vi "Two Backgate.vi"(0 "Sense":refnum<visa-resource-name>, 1 "Source":refnum<visa-resource-name>, 3 "Sense error in":errorcluster, 4 "Source error in":errorcluster, 6 "Input sweep":dbl[](array[numeric])) -> (8 "Read Time":dbl, 10 "BG Time Taken (s)":dbl, 11 "BackGate V":dbl[](array[numeric]), 12 "XY Graph":cluster{dbl[], "Ramp Pattern":dbl[]}(graph), 13 "Resistance":dbl[](array[numeric]), 14 "Sense Out":refnum<visa-resource-name>, 15 "Source Out":refnum<visa-resource-name>, 17 "Sense error out":errorcluster, 18 "Source error out":errorcluster)   [LabVIEW 2019, in "SMU.lvclass"]
uses:
  SMU.lvclass
  <instrlib>/Keithley 2450/Keithley 2450.lvlib
  <instrlib>/Keithley DMM6500 DAQ6500 Series/Keithley DMM6500 DAQ6500 Series.lvlib
panel:
  out "InitTime":dbl
  out "Total Time Taken (s) 2":dbl
  out "Sense Length":i32
  out "Current BG V":dbl
  out "Source buffer":string
  out "Current":dbl[](array[numeric])
  out "Voltage":dbl[](array[numeric])
  out "Sense buffer":string
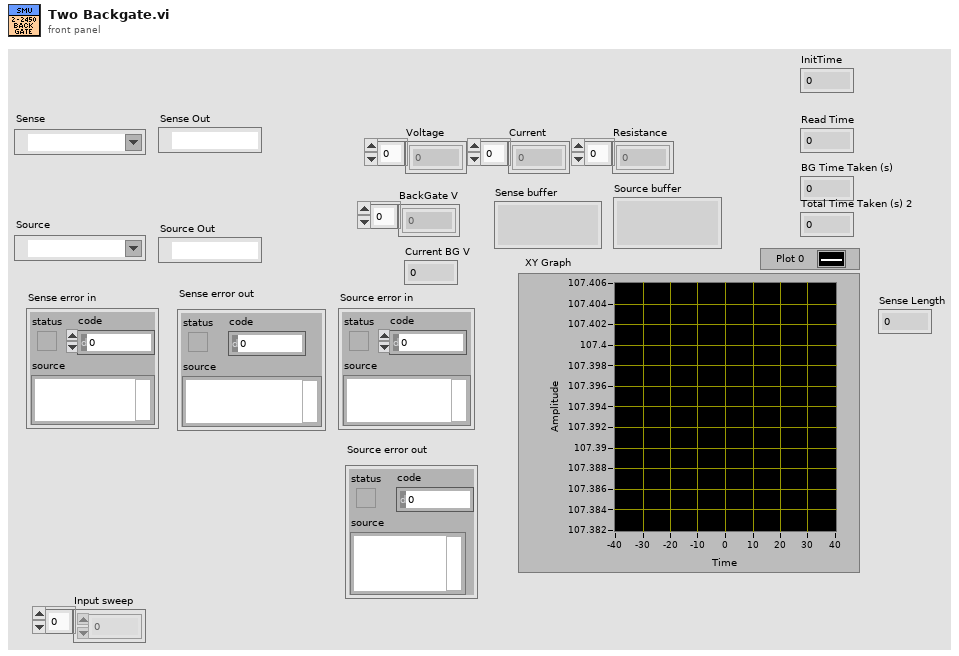
[diagram p1: front panel]
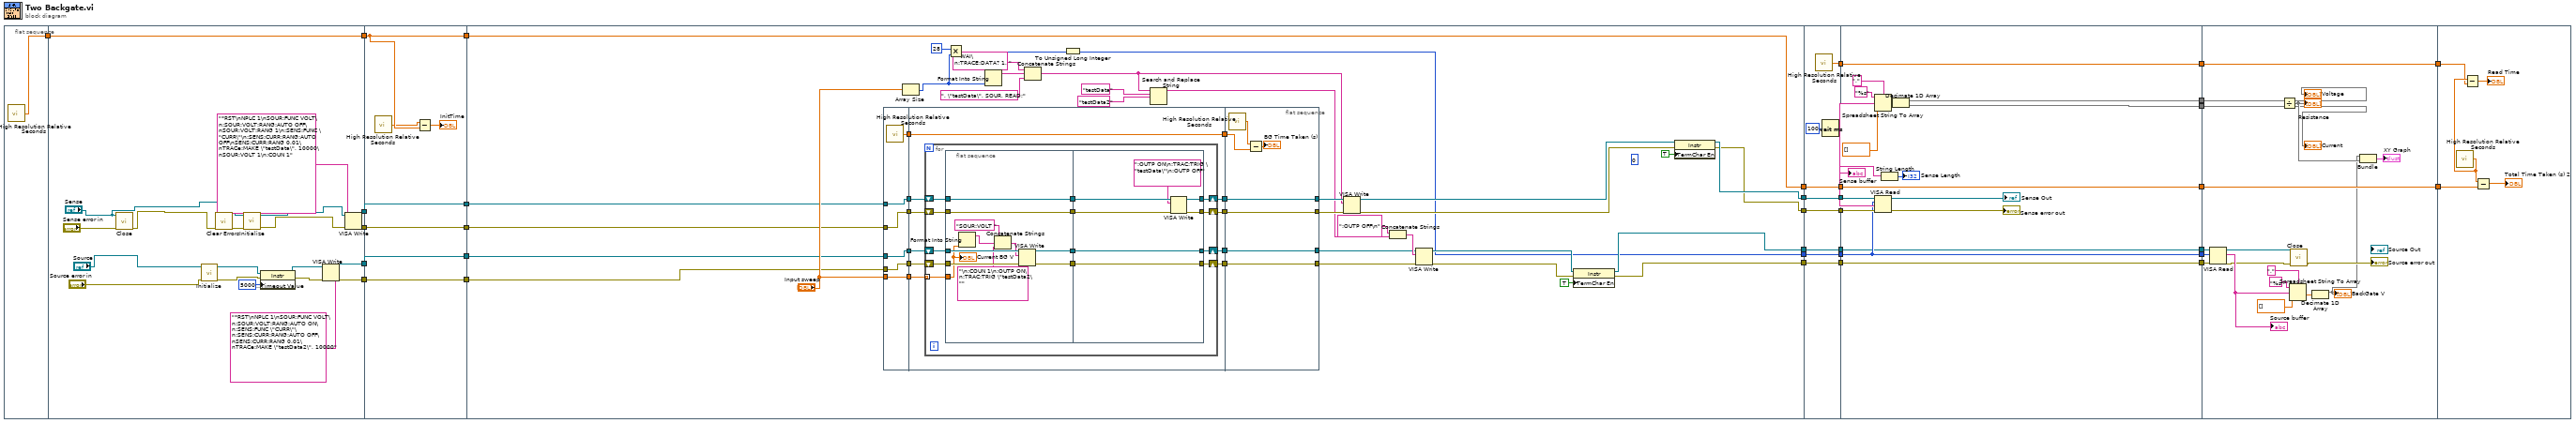
[diagram p0: block diagram]
diagram:
  n1 = flat-sequence {
    tunnel: [w34] -> w33
    tunnel: w33 -> [w54]
    tunnel: [w54] -> w20
    tunnel: [w41] -> w18
    tunnel: [w40] -> w16
    tunnel: [w39] -> w14
    tunnel: [w38] -> w12
    tunnel: w20 -> [w61]
    tunnel: [w61] -> w19
    tunnel: w18 -> [w60]
    tunnel: [w60] -> w17
    tunnel: w16 -> [w59]
    tunnel: [w59] -> w15
    tunnel: w14 -> [w58]
    tunnel: [w58] -> w13
    tunnel: w12 -> [w57]
    tunnel: [w57] -> w11
    tunnel: [w74] -> w32
    tunnel: w19 -> [w74]
    tunnel: w17 -> [w78]
    tunnel: w15 -> [w77]
    tunnel: w13 -> [w76]
    tunnel: w11 -> [w75]
    tunnel: [w63] -> w30
    tunnel: [w62] -> w28
    tunnel: [w64] -> w26
    tunnel: [w69] -> w23
    tunnel: [w68] -> w10
    tunnel: w32 -> [w167]
    tunnel: [w167] -> w31
    tunnel: w30 -> [w166]
    tunnel: [w166] -> w29
    tunnel: w28 -> [w165]
    tunnel: [w165] -> w27
    tunnel: w26 -> [w164]
    tunnel: [w164] -> w25
    tunnel: [w163] -> w24
    tunnel: w23 -> [w162]
    tunnel: [w162] -> w22
    tunnel: [w161] -> w21
    tunnel: w10 -> [w163]
    tunnel: w31 -> [w170]
    tunnel: [w170] -> w9
    tunnel: w29 -> [w175]
    tunnel: w27 -> [w174]
    tunnel: w25 -> [w173]
    tunnel: w24 -> [w179]
    tunnel: w22 -> [w178]
    tunnel: w21 -> [w176]
    tunnel: [w176] -> w7
    tunnel: [w175] -> w5
    tunnel: [w174] -> w4
    tunnel: [w173] -> w3
    tunnel: [w172] -> w2
    tunnel: [w171] -> w1
    tunnel: w9 -> [w202]
    tunnel: [w202] -> w8
    tunnel: w7 -> [w201]
    tunnel: [w201] -> w6
    tunnel: w5 -> [w194]
    tunnel: w4 -> [w193]
    tunnel: w3 -> [w192]
    tunnel: w2 -> [w188]
    tunnel: w1 -> [w187]
    tunnel: w8 -> [w206]
    tunnel: w6 -> [w204]
    frame #0 {
      n2 = call <vilib>:"High Resolution Relative Seconds.vi"() -> ("relative seconds"=w34:dbl)
    }
    frame #1 {
      n3 = call <instrlib>:"Close.vi"("error in (no error)"="Sense error in", "VISA resource name"="Sense") -> ("error out"=w47:errorcluster)  [unwired: 9 in]
      n4 = call <instrlib>:"Initialize.vi"("error in (no error)"="Source error in", "VISA resource name"="Source") -> ("error out"=w53:errorcluster, "VISA resource name out"=w50:refnum<visa-resource-name>)  [unwired: 8 in]
      n5 = call <vilib>:"Clear Errors.vi"("error in (no error)"=w47) -> ("error out"=w46:errorcluster)  [unwired: 5 in, 1 out]
      n6 = call <instrlib>:"Initialize.vi"("error in (no error)"=w46, "VISA resource name"="Sense") -> ("error out"=w37:errorcluster, "VISA resource name out"=w36:refnum<visa-resource-name>)  [unwired: 8 in]
      n7 = property class="Instr"(reference=w50, error in=w53, "General Settings:Timeout Value"=u32 5000) -> (reference out=w51:refnum<visa-resource-name>, error out=w52:errorcluster)
      n8 = VISA Write(VISA resource name=w51, write buffer="*RST\nNPLC 1\nSOUR:FUNC VOLT\n:SOUR:VOLT:RANG:AUTO ON\n:SENS:FUNC \"CURR\"\n:SENS:CURR:RANG:AUTO OFF\nSENS:CURR:RANG 0.01\nTRACe:MAKE \"testData2\", 10000", error in (no error)=w52) -> (VISA resource name out=w40:refnum<visa-resource-name>, error out=w41:errorcluster)  [unwired: 1 out]
      n9 = VISA Write(VISA resource name=w36, write buffer="*RST\nNPLC 1\nSOUR:FUNC VOLT\n:SOUR:VOLT:RANG:AUTO OFF\nSOUR:VOLT:RANG 1\n:SENS:FUNC \"CURR\"\n:SENS:CURR:RANG:AUTO OFF\nSENS:CURR:RANG 0.01\nTRACe:MAKE \"testData\", 10000\nSOUR:VOLT 1\n:COUN 1", error in (no error)=w37) -> (VISA resource name out=w38:refnum<visa-resource-name>, error out=w39:errorcluster)  [unwired: 1 out]
    }
    frame #2 {
      n10 = call <vilib>:"High Resolution Relative Seconds.vi"() -> ("relative seconds"=w55:dbl)
      n11 = Subtract(x=w55, y=w61) -> (x-y=→"InitTime":dbl)
    }
    frame #3 {
      (unwired) 0
      n12 = flat-sequence {
        tunnel: "Input sweep" -> [w111]
        tunnel: [w106] -> w105
        tunnel: [w107] -> w104
        tunnel: [w108] -> w103
        tunnel: [w109] -> w102
        tunnel: [w111] -> w101
        tunnel: [w110] -> w100
        tunnel: w78 -> [w109]
        tunnel: w77 -> [w108]
        tunnel: w76 -> [w107]
        tunnel: w75 -> [w106]
        tunnel: w105 -> [w121]
        tunnel: w104 -> [w120]
        tunnel: w103 -> [w117]
        tunnel: w102 -> [w116]
        tunnel: w101 -> [w113]
        tunnel: [w119] -> w99
        tunnel: [w118] -> w98
        tunnel: [w115] -> w97
        tunnel: [w114] -> w96
        tunnel: w100 -> [w112]
        tunnel: [w112] -> w95
        tunnel: [w158] -> w80
        tunnel: [w159] -> w79
        tunnel: [w153] -> w93
        tunnel: [w154] -> w94
        tunnel: w99 -> [w154]
        tunnel: w98 -> [w153]
        tunnel: w97 -> [w159]
        tunnel: w96 -> [w158]
        tunnel: w95 -> [w155]
        frame #0 {
          n13 = call <vilib>:"High Resolution Relative Seconds.vi"() -> ("relative seconds"=w110:dbl)
        }
        frame #1 {
          n14 = for {
            shift-right: [w133] -> w118
            shift-left: w121 -> [w134]
            shift-right: [w131] -> w119
            shift-left: w120 -> [w132]
            shift-right: [w126] -> w115
            shift-left: w117 -> [w128]
            shift-right: [w124] -> w114
            shift-left: w116 -> [w125]
            tunnel: w113 -> [w122] mode=indexing
            n15 = flat-sequence {
              tunnel: w132 -> [w144]
              tunnel: w134 -> [w145]
              tunnel: [w145] -> w130
              tunnel: [w144] -> w129
              tunnel: w128 -> [w143]
              tunnel: [w141] -> w127
              tunnel: w125 -> [w142]
              tunnel: [w140] -> w123
              tunnel: w122 -> [w136]
              tunnel: [w150] -> w133
              tunnel: [w148] -> w131
              tunnel: w130 -> [w152]
              tunnel: w129 -> [w149]
              tunnel: [w147] -> w126
              tunnel: w127 -> [w147]
              tunnel: [w146] -> w124
              tunnel: w123 -> [w146]
              frame #0 {
                n16 = Format Into String(w136) -> (resulting string=w137:string)  [unwired: 3 in, 1 out]
                n17 = Concatenate Strings("SOUR:VOLT ", w137, "\n:COUN 1\n:OUTP ON\n:TRAC:TRIG \"testData2\"") -> (w139:string)
                n18 = VISA Write(VISA resource name=w143, write buffer=w139, error in (no error)=w142) -> (VISA resource name out=w141:refnum<visa-resource-name>, error out=w140:errorcluster)  [unwired: 1 out]
                "Current BG V" <- w136
              }
              frame #1 {
                n19 = VISA Write(VISA resource name=w152, write buffer=":OUTP ON\n:TRAC:TRIG \"testData\"\n:OUTP OFF", error in (no error)=w149) -> (VISA resource name out=w150:refnum<visa-resource-name>, error out=w148:errorcluster)  [unwired: 1 out]
              }
            }
          }
        }
        frame #2 {
          n20 = call <vilib>:"High Resolution Relative Seconds.vi"() -> ("relative seconds"=w157:dbl)
          n21 = Subtract(x=w157, y=w155) -> (x-y=→"BG Time Taken (s)":dbl)
        }
      }
      n22 = Array Size(array="Input sweep") -> (size(s)=w82:i32)
      n23 = Multiply(x=28, y=w82) -> (x*y=w73:i32)
      n24 = Format Into String(w82) -> (resulting string=w92:string)  [unwired: 3 in, 1 out]
      n25 = Concatenate Strings("*WAI\n:TRACE:DATA? 1, ", w92, ", \"testData\", SOUR, READ;") -> (w87:string)
      n26 = To Unsigned Long Integer(number=w73) -> (unsigned 32bit integer=w62:u32)
      n27 = Search and Replace String(input string=w87, search string="testData", replace string="testData2" ("replace string (\"\")")) -> (result string=w84:string)  [unwired: 5 in, 3 out]
      n28 = VISA Write(VISA resource name=w93, write buffer=w87, error in (no error)=w94) -> (VISA resource name out=w71:refnum<visa-resource-name>, error out=w70:errorcluster)  [unwired: 1 out]
      n29 = Concatenate Strings(":OUTP OFF\n" ("string"), w84) -> (w88:string)
      n30 = VISA Write(VISA resource name=w79, write buffer=w88, error in (no error)=w80) -> (VISA resource name out=w66:refnum<visa-resource-name>, error out=w65:errorcluster)  [unwired: 1 out]
      n31 = property class="Instr"(reference=w66, error in=w65, "TermChar En"=TRUE ("Message Based Settings:Termination Character Enable")) -> (reference out=w64:refnum<visa-resource-name>, error out=w63:errorcluster)
      n32 = property class="Instr"(reference=w71, error in=w70, "TermChar En"=TRUE ("Message Based Settings:Termination Character Enable")) -> (reference out=w69:refnum<visa-resource-name>, error out=w68:errorcluster)
    }
    frame #4 {
      n33 = call <vilib>:"High Resolution Relative Seconds.vi"() -> ("relative seconds"=w161:dbl)
      n34 = Wait (ms)(milliseconds to wait=u32 100) -> ()  [unwired: 1 out]
    }
    frame #5 {
      n35 = VISA Read(VISA resource name=w178, byte count=w174, error in (no error)=w179) -> (VISA resource name out=→"Sense Out":refnum<visa-resource-name>, read buffer=w177:string, error out=→"Sense error out":errorcluster)  [unwired: 1 out]
      "Sense buffer" <- w177
      n36 = Spreadsheet String To Array(delimiter (Tab)=",", format string="%s", spreadsheet string=w177, array type (2D Dbl)=dbl[] []) -> (array=w183:dbl[])
      n37 = String Length(string=w177) -> (length=→"Sense Length":i32)
      n38 = Decimate 1D Array(w183) -> (w171:dbl[], w172:dbl[])
    }
    frame #6 {
      n39 = VISA Read(VISA resource name=w192, byte count=w193, error in (no error)=w194) -> (VISA resource name out=w186:refnum<visa-resource-name>, read buffer=w195:string, error out=w185:errorcluster)  [unwired: 1 out]
      "Source buffer" <- w195
      n40 = Divide(x=w187, y=w188) -> (x/y=w198:dbl[])
      "Resistance" <- w198
      n41 = Spreadsheet String To Array(delimiter (Tab)=",", format string="%s", spreadsheet string=w195, array type (2D Dbl)=dbl[] []) -> (array=w199:dbl[])
      n42 = call <instrlib>:"Close.vi"("error in (no error)"=w185, "VISA resource name"=w186) -> ("error out"=→"Source error out":errorcluster)  [unwired: 9 in]
      n43 = Decimate 1D Array(w199) -> (w197:dbl[])  [unwired: 1 out]
      "BackGate V" <- w197
      n44 = Bundle(w197, w198) -> (→"XY Graph":cluster{dbl[], dbl[]})  [unwired: 1 in]
      "Voltage" <- w187
      "Current" <- w188
    }
    frame #7 {
      n45 = call <vilib>:"High Resolution Relative Seconds.vi"() -> ("relative seconds"=w205:dbl)
      n46 = Subtract(x=w205, y=w204) -> (x-y=→"Read Time":dbl)
      n47 = Subtract(x=w205, y=w206) -> (x-y=→"Total Time Taken (s) 2":dbl)
    }
  }
